vi "V1fit.vi"(3 "output control":T2, 4 "data":T1, 5 "X":dbl[](array[numeric]), 6 "a":dbl[](array[numeric])) -> (0 "error out":errorcluster, 1 "f'(X,a)":dbl[][](array[numeric]), 2 "f(X,a)":dbl[](array[numeric]))   [LabVIEW 2018]
doc: "This template is the starting point for creating a model function to be passed to the Nonlinear Curve Fit.vi."
uses:
  <vilib>/gmath/NumericalOptimization/LM_output select.ctl
  <vilib>/gmath/NumericalOptimization/objective function data.ctl
  <vilib>/gmath/NI_Gmath.lvlib
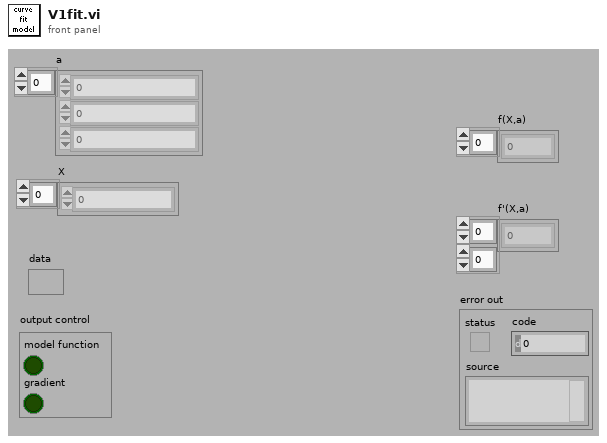
[diagram p1: front panel]
types:
  T1 = typedef "NI_Gmath.lvlib/objective function data.ctl" = variant
  T2 = typedef "NI_Gmath.lvlib/LM_output select.ctl" = cluster{"model function":bool, "gradient":bool}
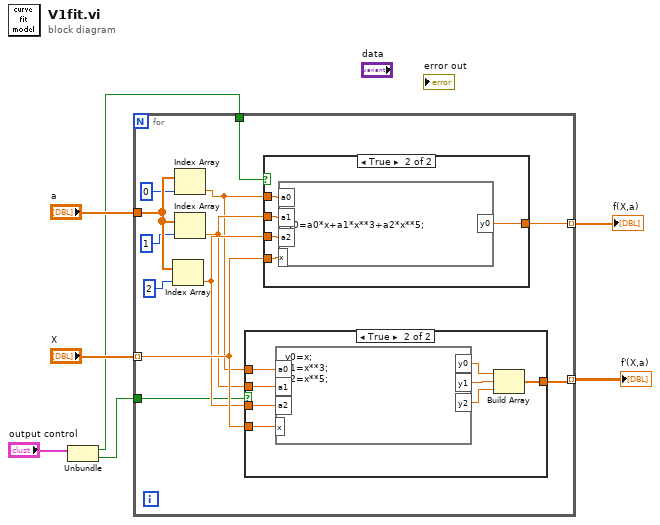
[diagram p0: block diagram]
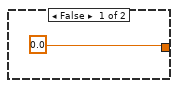
[diagram p2: hidden frame]
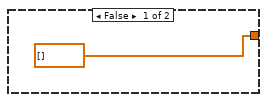
[diagram p3: hidden frame]
diagram:
  n1 = Unbundle("output control") -> ("model function"=w1:bool, "gradient"=w2:bool)
  n2 = for {
    tunnel: "a" -> [w17]
    tunnel: "X" -> [w19] mode=indexing
    tunnel: [w18] -> w5 mode=indexing
    tunnel: [w9] -> w4 mode=indexing
    tunnel: w2 -> [w10]
    tunnel: w1 -> [w8]
    n3 = Index Array(array=w17, index=2) -> (element=w13:dbl)
    n4 = Index Array(array=w17, index=0) -> (element=w11:dbl)
    n5 = Index Array(array=w17, index=1) -> (element=w12:dbl)
    n6 = case shown="True" w10 {
      tunnel: w19 -> [_ w34]
      tunnel: w13 -> [_ w33]
      tunnel: w12 -> [_ w32]
      tunnel: w11 -> [_ w31]
      tunnel: [dbl[] [] w27] -> w9
      frame False {
      }
      frame True {
        n7 = formula code="y0=x;\ny1=x**3;\ny2=x**5;"("x"=w34, "a0"=w31, "a1"=w32, "a2"=w33) -> ("y0"=w28:dbl, "y1"=w29:dbl, "y2"=w30:dbl)
        n8 = Build Array(w28, w29, w30) -> (w27:dbl[])
      }
    }
    n9 = case shown="True" w8 {
      tunnel: w19 -> [_ w25]
      tunnel: [0.0 w24] -> w18
      tunnel: w13 -> [_ w23]
      tunnel: w12 -> [_ w22]
      tunnel: w11 -> [_ w21]
      frame False {
      }
      frame True {
        n10 = formula code="y0=a0*x+a1*x**3+a2*x**5;"("x"=w25, "a0"=w21, "a2"=w23, "a1"=w22) -> ("y0"=w24:dbl)
      }
    }
  }
  "f(X,a)" <- w5
  "f'(X,a)" <- w4
